vi "Generate Month Load SQL Query.vi"(8 "error in (no error)":errorcluster, 10 "SQL Date":string, 11 "Statement in":refnum<class "Statement.lvclass">) -> (0 "error out":errorcluster, 2 "SQL Query":string, 3 "Statement out":refnum<class "Statement.lvclass">)   [LabVIEW 2018, in "Statement.lvclass"]
uses:
  Statement.lvclass
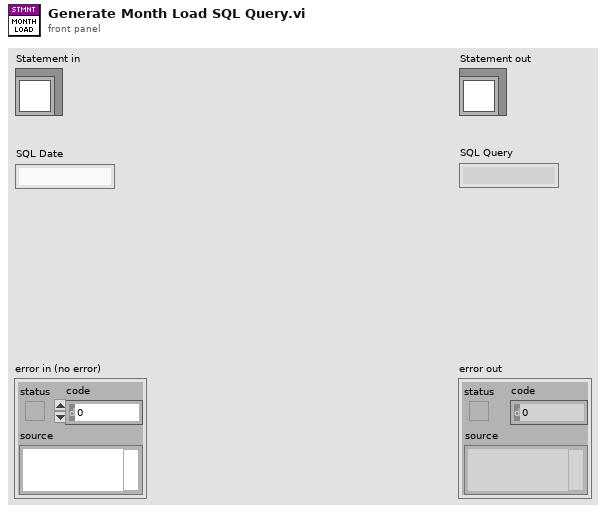
[diagram p1: front panel]
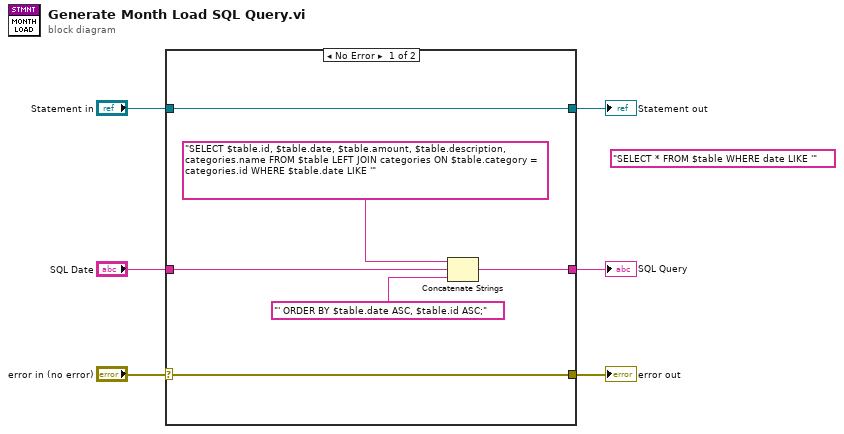
[diagram p0: block diagram]
diagram:
  (unwired) "SELECT * FROM $table WHERE date LIKE '"
  n1 = case shown="No Error" "error in (no error)" {
    selector: "error in (no error)" -> [w11 w14]
    tunnel: [w11 w14] -> w5
    tunnel: [w12 w13] -> w3
    tunnel: "Statement in" -> [w12 w13]
    tunnel: "SQL Date" -> [w10 _]
    tunnel: [w8 _] -> w1
    frame No Error {
      n2 = Concatenate Strings("SELECT $table.id, $table.date, $table.amount, $table.description, categories.name FROM $table LEFT JOIN categories ON $table.category = categories.id WHERE $table.date LIKE '", w10, "' ORDER BY $table.date ASC, $table.id ASC;" ("string")) -> (w8:string)
    }
    frame Error {
    }
  }
  "error out" <- w5
  "Statement out" <- w3
  "SQL Query" <- w1
